vi "VISA AMI430 Write-Read.vi"(8 "error in (no error)":errorcluster {"code" format="%.0x"}, 9 "Command String":string="*IDN?", 10 "Action":enum16{"Write", "Read", "Write & Read"}(ring)=enum."Write & Read", 11 "VISA resource name":refnum<visa-resource-name>) -> (0 "error out":errorcluster, 1 "Timeout?":bool, 2 "Response string":string, 3 "dup VISA Session":refnum<visa-resource-name>)   [LabVIEW 2025]
doc: "Author: Scott Hannahs <sth@magnet.fsu.edu>\n\nThis software is licensed for use under the “MIT License\"\nCopyright (c) 2025 Scott Hannahs, sth@sth@magnet.sthnet.net\n\nPermission is hereby granted, free of charge, to any person obtaining a copy of this software and associated documentation files (the \"Software\"), to deal in the Software without restriction, including without limitation the rights to use, copy, modify, merge, publish, distribute, sublicense, and/or sell copies of the Software, and to permit persons to whom the Software is furnished to do so, subject to the following conditions: The above copyright notice and this permission notice shall be included in all copies or substantial portions of the Software.\n\nTHE SOFTWARE IS PROVIDED \"AS IS\", WITHOUT WARRANTY OF ANY KIND, EXPRESS OR IMPLIED, INCLUDING BUT NOT LIMITED TO THE WARRANTIES OF MERCHANTABILITY, FITNESS FOR A PARTICULAR PURPOSE AND NONINFRINGEMENT. IN NO EVENT SHALL THE AUTHORS OR COPYRIGHT HOLDERS BE LIABLE FOR ANY CLAIM, DAMAGES OR OTHER LIABILITY, WHETHER IN AN ACTION OF CONTRACT, TORT OR OTHERWISE, ARISING FROM, OUT OF OR IN CONNECTION WITH THE SOFTWARE OR THE USE OR OTHER DEALINGS IN THE SOFTWARE."
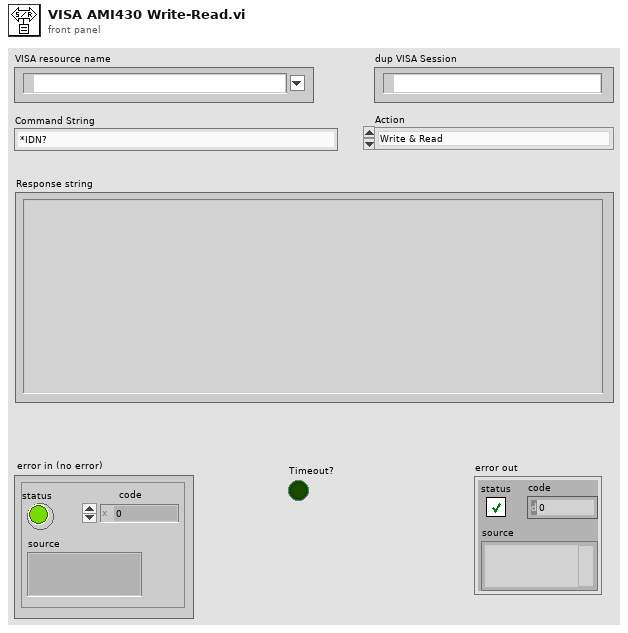
[diagram p1: front panel]
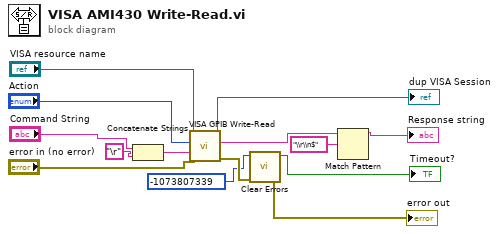
[diagram p0: block diagram]
diagram:
  n1 = Concatenate Strings("Command String", "\r") -> (w3:string)
  n2 = call "VISA GPIB Write-Read.vi"("error in (no error)"="error in (no error)", "Command"=w3, "Action"="Action", "VISA resource name"="VISA resource name") -> ("error out"=w10:errorcluster, "String Returned"=w7:string, "dup VISA Session"=→"dup VISA Session":refnum<visa-resource-name>)  [unwired: 4 in, 1 out]
  n3 = call <vilib>:"Clear Errors.vi"("error in (no error)"=w10, "specific error code to clear (0: all)"=-1073807339) -> ("error out"=→"error out":errorcluster, "specific error cleared?"=→"Timeout?":bool)  [unwired: 4 in]
  n4 = Match Pattern(string=w7, regular expression="\\r\\n$") -> (before substring=→"Response string":string)  [unwired: 1 in, 3 out]
